vi "Inspect Call.vi"(8 "Error in":errorcluster, 9 "Msg in":refnum<class "Msg.lvclass">, 11 "TEMPLATE Actor in":refnum<class "TEMPLATE Actor.lvclass">) -> (0 "Error out":errorcluster, 1 "Msg out":refnum<class "Msg.lvclass">, 2 "Proceed To Execute Or Recurse":bool=TRUE, 3 "TEMPLATE Actor out":refnum<class "TEMPLATE Actor.lvclass">)   [LabVIEW 2020, in "_Template.lvlib" / "Templates.lvlib" / "TEMPLATE jettl Actor.lvlib" / "TEMPLATE Actor.lvlib" / "TEMPLATE Actor.lvclass"]
uses:
  TEMPLATE Actor.lvclass
  jettl/jettl/Msg/Msg.lvclass
  TEMPLATE Actor.lvclass/TEMPLATE Actor.ctl
  jettl/jettl/Actor/Actor.lvclass
panel:
  # "This front panel should not be manipulated."
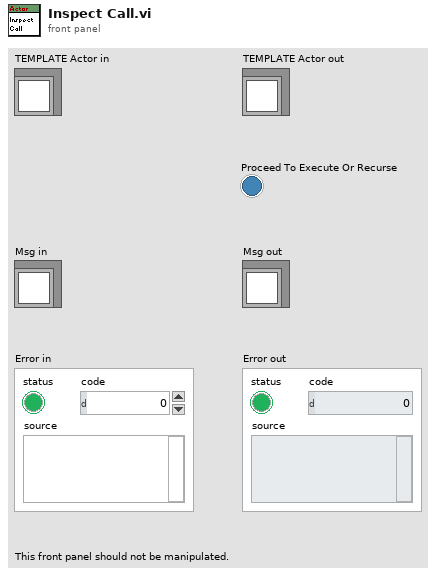
[diagram p1: front panel]
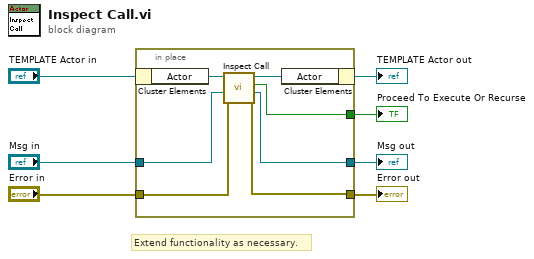
[diagram p0: block diagram]
diagram:
  # "Extend functionality as necessary."
  n1 = in-place {
    in-place-border: "Error in" -> [w12]
    in-place-border: [w8] -> w6
    in-place-border: [w10] -> w5
    in-place-border: "Msg in" -> [w13]
    in-place-border: [w9] -> w1
    n2 = in-place-cluster #1("TEMPLATE Actor in") -> ("Actor"=w14:refnum<class "Actor.lvclass">)
    n3 = call-dynamic "Inspect Call.vi"("Error in"=w12, "Msg in"=w13, "Actor in"=w14) -> ("Error out"=w8:errorcluster, "Msg out"=w9:refnum<class "Msg.lvclass">, "Proceed To Execute Or Recurse"=w10:bool, "Actor out"=w11:refnum<class "Actor.lvclass">)  [unwired: 5 in]
    n4 = in-place-cluster #1("Actor"=w11) -> (→"TEMPLATE Actor out":refnum<class "TEMPLATE Actor.lvclass">)
  }
  "Proceed To Execute Or Recurse" <- w5
  "Error out" <- w6
  "Msg out" <- w1
